vi "FRCts20_Backend_Test_EventRoot_POST.vi"(8 "error in (no error)":errorcluster, 11 "EventRoot In":T1) -> (0 "error out":errorcluster, 1 "Time (ms)":u32, 2 "Status":string, 3 "Events":T1, 5 "Success":bool)   [LabVIEW 2014, in "FRCts20_Backend_TestCode.lvlib"]
uses:
  FRCts20_Backend_TestCode.lvlib
  FRCts20_Backend_API/FRCts20_Backend_API_EventRoot.vi
  FRCts20_Backend_API/FRCts20_Backend_API_Command_EventRoot.ctl
  FRCts20_Backend_API/FRCts20_Backend_API_EventRoot.ctl
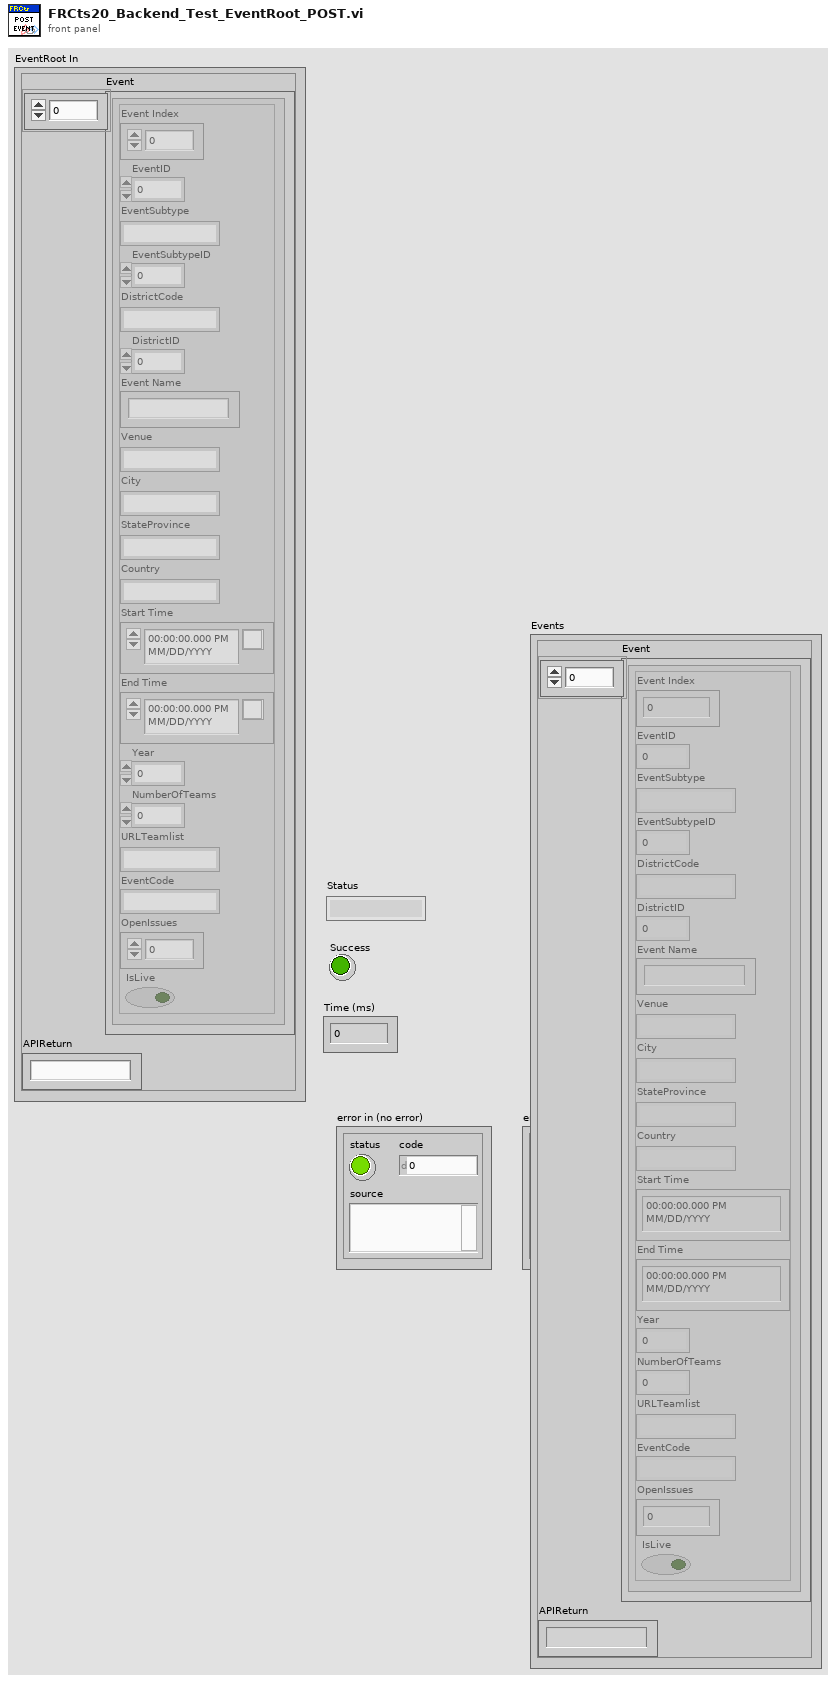
[diagram p1: front panel]
types:
  T1 = typedef "FRCts20_Backend_API.lvlib/FRCts20_Backend_API_EventRoot.ctl" = cluster{"Event":cluster{"Event Index":u32, "EventID":u32, "EventSubtype":string, "EventSubtypeID":u32, "DistrictCode":string, "DistrictID":u32, "Event Name":string, "Venue":string, "City":string, "StateProvince":string, "Country":string, "Start Time":timestamp, "End Time":timestamp, "Year":u32, "NumberOfTeams":u32, "URLTeamlist":string, "EventCode":string, "OpenIssues":u8, "IsLive":bool}[], "APIReturn":string}
  T2 = typedef "FRCts20_Backend_API.lvlib/FRCts20_Backend_API_Command_EventRoot.ctl" = string
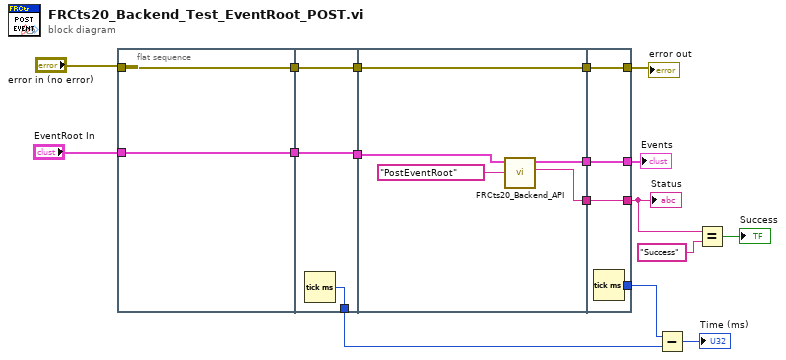
[diagram p0: block diagram]
diagram:
  n1 = flat-sequence {
    tunnel: "error in (no error)" -> [w19]
    tunnel: [w19] -> w17
    tunnel: [w18] -> w3
    tunnel: "EventRoot In" -> [w18]
    tunnel: [w22] -> w6
    tunnel: [w21] -> w16
    tunnel: w17 -> [w21]
    tunnel: w3 -> [w20]
    tunnel: [w20] -> w1
    tunnel: [w27] -> w15
    tunnel: w16 -> [w27]
    tunnel: [w26] -> w14
    tunnel: [w25] -> w13
    tunnel: w1 -> [w23]
    tunnel: [w31] -> w7
    tunnel: [w30] -> w9
    tunnel: w15 -> [w30]
    tunnel: [w29] -> w4
    tunnel: w14 -> [w29]
    tunnel: [w28] -> w5
    tunnel: w13 -> [w28]
    frame #0 {
    }
    frame #1 {
      n2 = Tick Count (ms)() -> (millisecond timer value=w22:u32)
    }
    frame #2 {
      n3 = call-poly "FRCts20_Backend_API.vi"("Message"=T2 "PostEventRoot", "EventRoot In"=w23) -> ("Status"=w25:string, "EventRoot Out"=w26:T1)  [unwired: 7 in, 1 out]
    }
    frame #3 {
      n4 = Tick Count (ms)() -> (millisecond timer value=w31:u32)
    }
  }
  n5 = Subtract(x=w7, y=w6) -> (x-y=→"Time (ms)":u32)
  n6 = Equal?(x=w5, y="Success") -> (x = y?=→"Success":bool)
  "Status" <- w5
  "error out" <- w9
  "Events" <- w4
